vi "Доп Код.vi"(0 "C7":bool, 1 "B":T2) -> (2 "b":T1)   [LabVIEW 2017]
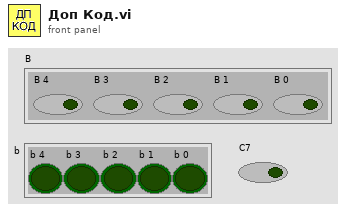
[diagram p1: front panel]
types:
  T1 = cluster{"b 4":bool, "b 3":bool, "b 2":bool, "b 1":bool, "b 0":bool}
  T2 = cluster{"B 4":bool, "B 3":bool, "B 2":bool, "B 1":bool, "B 0":bool}
  T3 = cluster{"SO":bool, "SO":bool, "SO":bool, "SO":bool, "SO":bool}
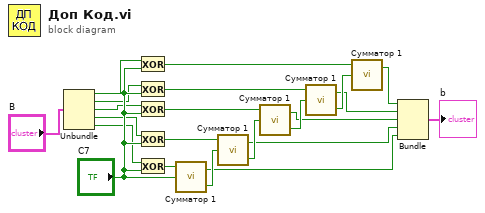
[diagram p0: block diagram]
diagram:
  n1 = Unbundle("B") -> ("B 4"=w11:bool, "B 3"=w10:bool, "B 2"=w9:bool, "B 1"=w8:bool, "B 0"=w7:bool)
  n2 = Exclusive Or(1:"C7", 2:w11) -> (0:w13:bool)
  n3 = Exclusive Or(1:"C7", 2:w10) -> (0:w15:bool)
  n4 = Exclusive Or(1:"C7", 2:w9) -> (0:w17:bool)
  n5 = Exclusive Or(1:"C7", 2:w8) -> (0:w20:bool)
  n6 = Exclusive Or(1:"C7", 2:w7) -> (0:w22:bool)
  n7 = call "Сумматор 1.vi"("B"="C7", "A"=w22) -> ("S1"=w19:bool, "SO"=w2:bool)  [unwired: 1 in]
  n8 = call "Сумматор 1.vi"("B"=w19, "A"=w20) -> ("S1"=w18:bool, "SO"=w3:bool)  [unwired: 1 in]
  n9 = call "Сумматор 1.vi"("B"=w18, "A"=w17) -> ("S1"=w16:bool, "SO"=w4:bool)  [unwired: 1 in]
  n10 = call "Сумматор 1.vi"("B"=w16, "A"=w15) -> ("S1"=w14:bool, "SO"=w5:bool)  [unwired: 1 in]
  n11 = call "Сумматор 1.vi"("B"=w14, "A"=w13) -> ("SO"=w6:bool)  [unwired: 1 in, 1 out]
  n12 = Bundle("SO"=w6, "SO"=w5, "SO"=w4, "SO"=w3, "SO"=w2) -> (→"b":T3)  [unwired: 1 in]
